vi "Example of fetch git 7-digi hash somewhere.vi"() -> ()   [LabVIEW 2016]
panel:
  in  "Git repo path":path=path "C:/"
  out "Fetch error?":bool
  out "error out":errorcluster
  out "Hash:":string
  # "Run the VI to get abbreviated hash with git branch command"
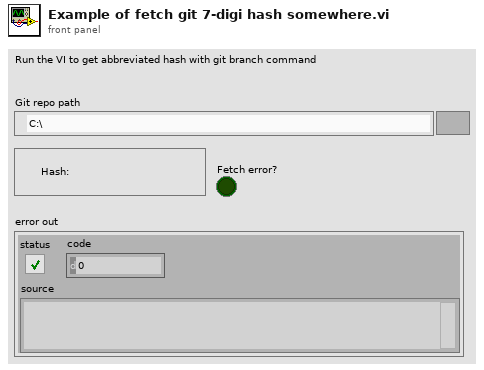
[diagram p1: front panel]
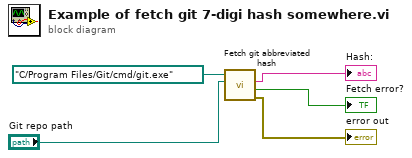
[diagram p0: block diagram]
diagram:
  n1 = call "Fetch git abbreviated hash.vi"("git repo path"="Git repo path", "git.exe path"=path "C:/Program Files/Git/cmd/git.exe") -> ("error out"=→"error out":errorcluster, "Fetch error?"=→"Fetch error?":bool, "Abbreviated hash"=→"Hash:":string)  [unwired: 6 in, 1 out]
